vi "Panel Centre Position.vi"(10 "Panel size":cluster{"Height":i16, "Width":i16}, 11 "Monitor Bounds":T1) -> (3 "Position":cluster{"Top":i16, "Left":i16})   [LabVIEW 2014]
uses:
  <vilib>/Utility/miscctls.llb/LVRectTypeDef.ctl
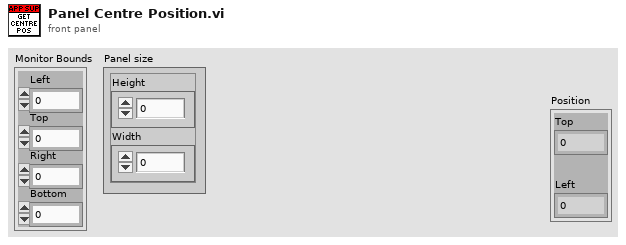
[diagram p1: front panel]
types:
  T1 = typedef "LVRectTypeDef.ctl" = cluster{"Left":i16, "Top":i16, "Right":i16, "Bottom":i16}
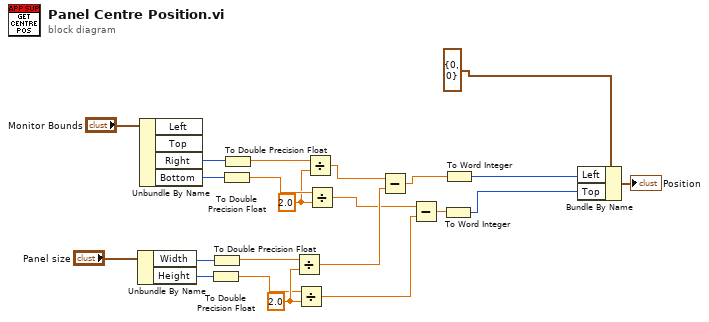
[diagram p0: block diagram]
diagram:
  w15 = 2.0 ("y")
  w17 = 2.0 ("y")
  n1 = Unbundle By Name("Panel size") -> ("Width"=w12:i16, "Height"=w11:i16)
  n2 = Unbundle By Name("Monitor Bounds") -> ("Right"=w21:i16, "Bottom"=w20:i16)  [unwired: 2 out]
  n3 = To Double Precision Float(number=w11) -> (double precision float=w14:dbl)
  n4 = To Double Precision Float(number=w12) -> (double precision float=w13:dbl)
  n5 = To Double Precision Float(number=w20) -> (double precision float=w18:dbl)
  n6 = To Double Precision Float(number=w21) -> (double precision float=w19:dbl)
  n7 = Divide(x=w13, y=w15) -> (x/y=w9:dbl)
  n8 = Divide(x=w14, y=w15) -> (x/y=w7:dbl)
  n9 = Divide(x=w19, y=w17) -> (x/y=w10:dbl)
  n10 = Divide(x=w18, y=w17) -> (x/y=w8:dbl)
  n11 = Subtract(x=w10, y=w9) -> (x-y=w5:dbl)
  n12 = Subtract(x=w8, y=w7) -> (x-y=w4:dbl)
  n13 = To Word Integer(number=w4) -> (16bit integer=w3:i16)
  n14 = To Word Integer(number=w5) -> (16bit integer=w2:i16)
  n15 = Bundle By Name(cluster=cluster{"Top":i16, "Left":i16} {"Top"=0, "Left"=0} ("Position"), "Left"=w2, "Top"=w3) -> (→"Position":cluster{"Top":i16, "Left":i16})
